vi "read_attributes.vi"(8 "error in (no error)":errorcluster, 11 "NearestCentroid in":refnum<class "NearestCentroid.lvclass">) -> (0 "error out":errorcluster, 2 "attributes":T1, 3 "NearestCentroid out":refnum<class "NearestCentroid.lvclass">)   [LabVIEW 2020, in "NearestCentroid.lvclass"]
uses:
  NearestCentroid.lvclass
  Controls/nearest_centroid_attributes.ctl
  NearestCentroid.lvclass/NearestCentroid.ctl
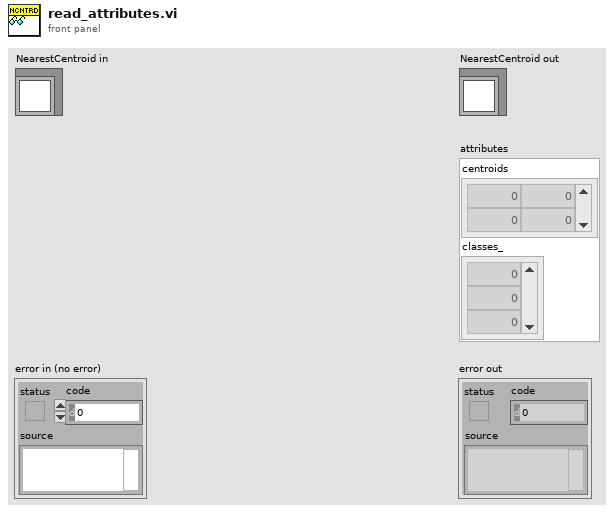
[diagram p1: front panel]
types:
  T1 = typedef "nearest_centroid_attributes.ctl" = cluster{"centroids":dbl[][], "classes_":dbl[]}
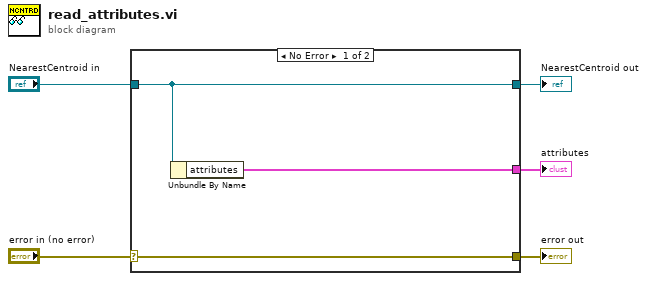
[diagram p0: block diagram]
diagram:
  n1 = case shown="No Error" "error in (no error)" {
    selector: "error in (no error)" -> [w8 w9]
    tunnel: [w8 w9] -> w4
    tunnel: [w7 w10] -> w2
    tunnel: "NearestCentroid in" -> [w7 w10]
    tunnel: [w6 _] -> w1
    frame No Error {
      n2 = Unbundle By Name(w7) -> ("attributes"=w6:T1)
    }
    frame Error {
    }
  }
  "error out" <- w4
  "NearestCentroid out" <- w2
  "attributes" <- w1
